vi "Add Hardware.vi"(8 "error in (no error)":errorcluster, 10 "Hardware.lvclass":refnum<class "Hardware.lvclass">, 11 "Controller in":refnum<class "Controller.lvclass">) -> (0 "error out":errorcluster, 3 "Controller out":refnum<class "Controller.lvclass">)   [LabVIEW 2017, in "Controller Actor.lvlib" / "Controller.lvclass"]
uses:
  Controller.lvclass
  C:/Program Files (x86)/National Instruments/LabVIEW 2017/vi.lib/ActorFramework/Actor/Actor.lvclass
  Hardware/Hardware.lvclass
  Controller.lvclass/Controller.ctl
  <userlib>/Configuration Dialog Actor/Configuration.lvclass/Configuration.ctl
  Hardware/Hardware.lvclass/Hardware.ctl
  <vilib>/ActorFramework/Actor/Actor.lvclass/Actor.ctl
  <vilib>/ActorFramework/Message Enqueuer/Message Enqueuer.lvclass/Message Enqueuer.ctl
  <vilib>/ActorFramework/Message Enqueuer/Init from Existing Queue.vi
  Hardware/HW Config/HW Configuration.lvclass
  C:/Program Files (x86)/National Instruments/LabVIEW 2017/user.lib/Configuration Dialog Actor/Configuration.lvclass
  <vilib>/Utility/LVClass/Get LV Class Path.vi
  <userlib>/_OpenG.lib/file/file.llb/Strip Path Extension__ogtk.vi
  <userlib>/_OpenG.lib/file/file.llb/Strip Path Extension - String__ogtk.vi
  <userlib>/Configuration Dialog Actor/Configuration.lvclass
  <vilib>/ActorFramework/Message Enqueuer/Message Enqueuer.lvclass
  Messages/Log Status/Log Status.lvclass
  <vilib>/ActorFramework/Actor/Actor.lvclass
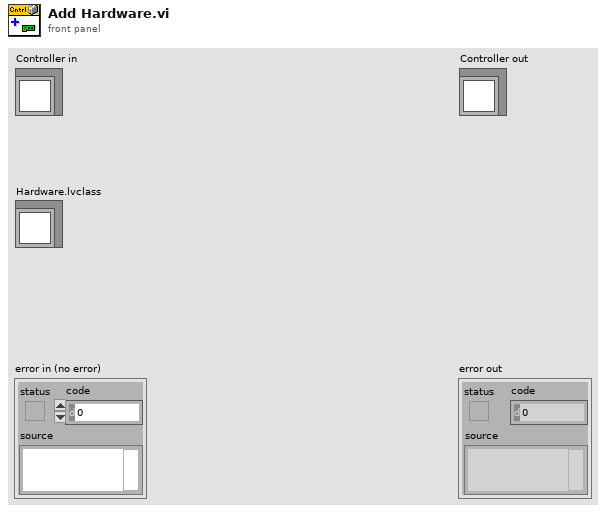
[diagram p1: front panel]
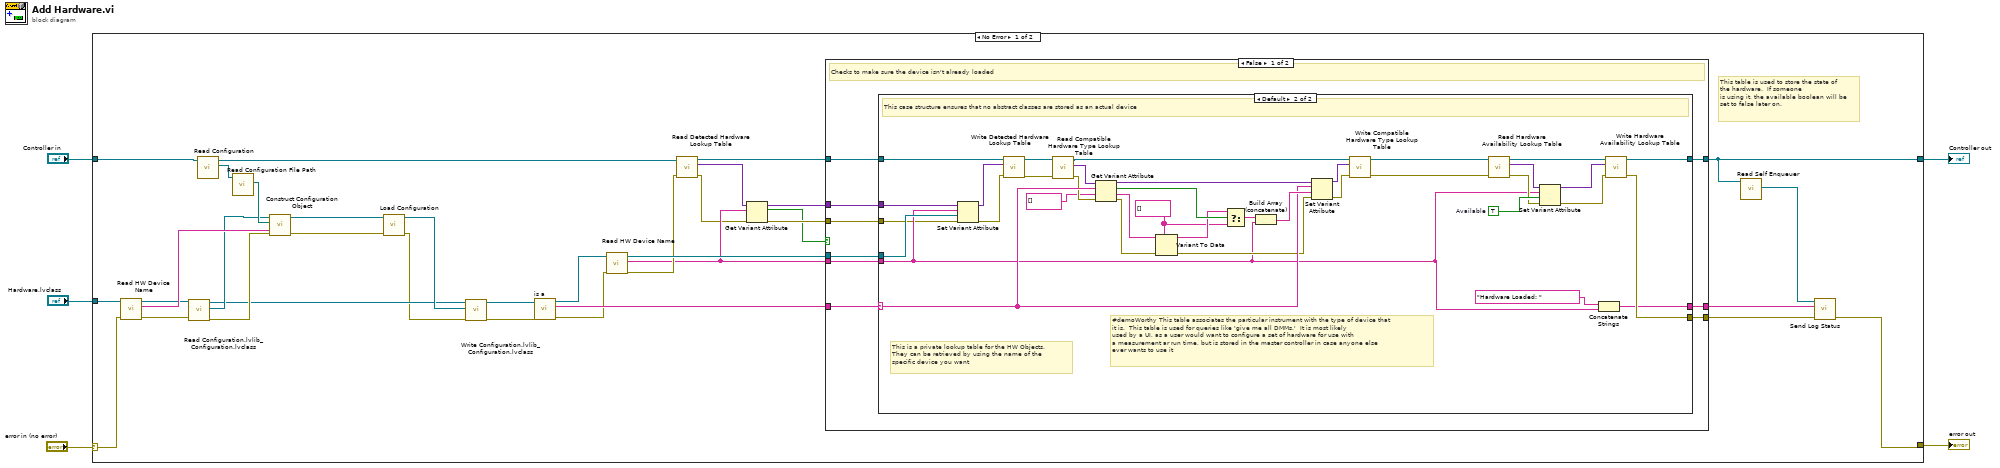
[diagram p0: block diagram]
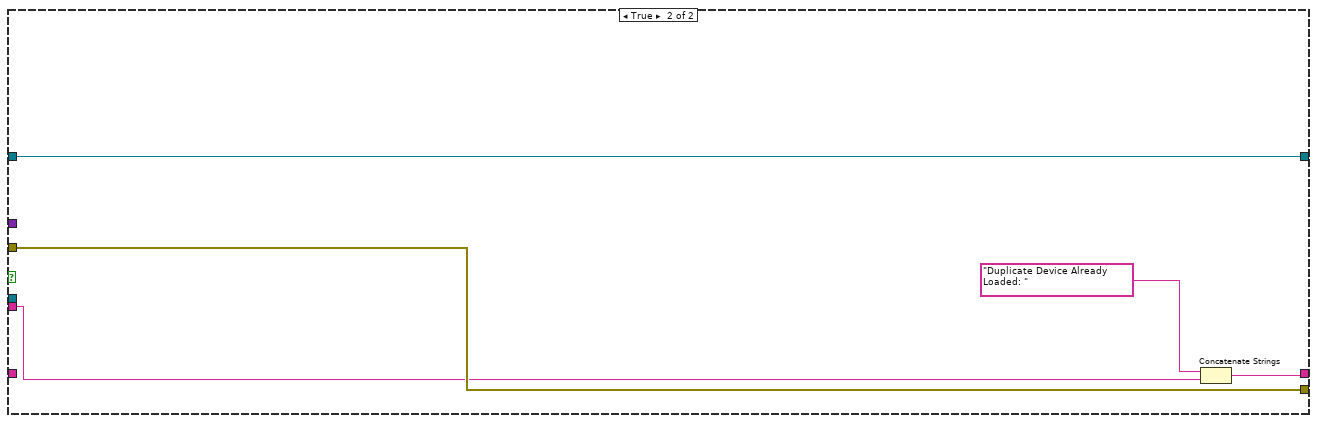
[diagram p3: hidden frame]
diagram:
  n1 = case shown="No Error" "error in (no error)" {
    selector: "error in (no error)" -> [w6 w94]
    tunnel: [w38 w94] -> w4
    tunnel: [w26 w93] -> w2
    tunnel: "Controller in" -> [w19 w93]
    tunnel: "Hardware.lvclass" -> [w17 _]
    frame No Error {
      # "This table is used to store the state of the hardware.  If someone\nis using it, the available boolean will be set to false later on."
      n2 = call "Read HW Device Name.vi"("error in (no error)"=w6, "Analog in"=w17) -> ("error out"=w11:errorcluster, "Device Name"=w16:string, "Analog out"=w13:refnum<class "Hardware.lvclass">)  [unwired: 7 in]
      n3 = call-dynamic "Read Configuration.lvlib_Configuration.lvclass.vi"("error in (no error)"=w11, "Hardware in"=w13) -> ("error out"=w10:errorcluster, "Hardware.lvlib:HW Configuration.lvclass"=w14:refnum<class "HW Configuration.lvclass">, "Hardware out"=w9:refnum<class "Hardware.lvclass">)  [unwired: 7 in]
      n4 = call "Read Configuration.vi"("Controller in"=w19) -> ("Configuration.lvlib:Configuration.lvclass"=w21:refnum<class "Configuration.lvclass">, "Controller out"=w18:refnum<class "Controller.lvclass">)  [unwired: 8 in, 1 out]
      n5 = call <userlib>:"Read Configuration File Path.vi"("Configuration in"=w21) -> ("Configuration File Path"=w20:path)  [unwired: 8 in, 2 out]
      n6 = call <userlib>:"Construct Configuration Object.vi"("Group Name"=w16, "error in (no error)"=w10, "Configuration File Path"=w20, "Configuration in"=w14) -> ("error out"=w22:errorcluster, "Configuration out"=w23:refnum<class "HW Configuration.lvclass">)  [unwired: 4 in, 2 out]
      n7 = call <userlib>:"Load Configuration.vi"("error in (no error)"=w22, "Configuration in"=w23) -> ("error out"=w8:errorcluster, "Configuration out"=w15:refnum<class "HW Configuration.lvclass">)  [unwired: 7 in, 1 out]
      n8 = call-dynamic "Write Configuration.lvlib_Configuration.lvclass.vi"("error in (no error)"=w8, "Hardware.lvlib:HW Configuration.lvclass"=w15, "Hardware in"=w9) -> ("error out"=w7:errorcluster, "Hardware out"=w12:refnum<class "Hardware.lvclass">)  [unwired: 7 in]
      n9 = call-dynamic "is a.vi"("error in (no error)"=w7, "Hardware in"=w12) -> ("error out"=w35:errorcluster, "is a"=w39:string, "Hardware out"=w36:refnum<class "Hardware.lvclass">)  [unwired: 7 in]
      n10 = call "Read HW Device Name.vi"("error in (no error)"=w35, "Analog in"=w36) -> ("error out"=w33:errorcluster, "Device Name"=w30:string, "Analog out"=w37:refnum<class "Hardware.lvclass">)  [unwired: 7 in]
      n11 = call "Read Detected Hardware Lookup Table.vi"("error in (no error)"=w33, "Controller in"=w18) -> ("error out"=w29:errorcluster, "Detected Hardware Lookup Table"=w32:variant, "Controller out"=w34:refnum<class "Controller.lvclass">)  [unwired: 7 in]
      n12 = Get Variant Attribute(Variant=w32, name=w30, error in=w29) -> (duplicate Variant=w31:variant, found=w24:bool, error out=w28:errorcluster)  [unwired: 1 in, 1 out]
      n13 = case shown="False" w24 {
        tunnel: w39 -> [w48 _]
        tunnel: [w47 w91] -> w38
        tunnel: w37 -> [w46 _]
        tunnel: w34 -> [w45 w92]
        tunnel: w31 -> [w44 _]
        tunnel: w30 -> [w43 w88]
        tunnel: w28 -> [w42 w91]
        tunnel: [w41 w92] -> w26
        tunnel: [w40 w89] -> w25
        frame False {
          # "Checks to make sure the device isn't already loaded"
          n14 = case shown="Default" w48 {
            selector: w48 -> [_ w69]
            tunnel: w45 -> [w50 w55]
            tunnel: [w50 w70] -> w41
            tunnel: [w49 w52] -> w47
            tunnel: w46 -> [_ w57]
            tunnel: w43 -> [_ w56]
            tunnel: w44 -> [_ w54]
            tunnel: w42 -> [w49 w53]
            tunnel: [_ w51] -> w40
            frame "Abstract Class" {
            }
            frame Default {
              w75 = TRUE  # Available
              w81 = string[] []
              # "This is a private lookup table for the HW Objects.  \nThey can be retrieved by using the name of the\nspecific device you want"
              # "#demoWorthy This table associates the particular instrument with the type of device that\nit is.  This table is used for queries like 'give me all DMMs.'  It is most likely\nused by a UI, as a user would want to configure a set of hardware for use with\na measurement ar run time, but is stored in the master controller in case anyone else\never wants to use it"
              # "This case structure ensures that no abstract classes are stored as an actual device"
              n15 = Set Variant Attribute(Variant=w54, name=w56, value=w57, error in=w53) -> (Variant out=w87:variant, error out=w66:errorcluster)  [unwired: 1 out]
              n16 = call "Write Detected Hardware Lookup Table.vi"("error in (no error)"=w66, "Detected Hardware Lookup Table"=w87, "Controller in"=w55) -> ("error out"=w67:errorcluster, "Controller out"=w79:refnum<class "Controller.lvclass">)  [unwired: 7 in]
              n17 = call "Read Compatible Hardware Type Lookup Table.vi"("error in (no error)"=w67, "Controller in"=w79) -> ("error out"=w68:errorcluster, "Compatible Hardware Type Lookup Table"=w76:variant, "Controller out"=w78:refnum<class "Controller.lvclass">)  [unwired: 7 in]
              n18 = Get Variant Attribute(Variant=w76, name=w69, default value (empty Variant)=string[] [], error in=w68) -> (duplicate Variant=w80:variant, found=w84:bool, value=w86:string[], error out=w65:errorcluster)
              n19 = Variant To Data(error in=w65, type=w81, Variant=w86) -> (data=w82:string[], error out=w64:errorcluster)
              n20 = Select(t=w82, s=w84, f=w81) -> (s? t:f=w83:string[])
              n21 = Build Array (concatenate)(w83, w56) -> (w85:string[])
              n22 = Set Variant Attribute(Variant=w80, name=w69, value=w85, error in=w64) -> (Variant out=w77:variant, error out=w63:errorcluster)  [unwired: 1 out]
              n23 = call "Write Compatible Hardware Type Lookup Table.vi"("error in (no error)"=w63, "Compatible Hardware Type Lookup Table"=w77, "Controller in"=w78) -> ("error out"=w62:errorcluster, "Controller out"=w74:refnum<class "Controller.lvclass">)  [unwired: 7 in]
              n24 = call "Read Hardware Availability Lookup Table.vi"("error in (no error)"=w62, "Controller in"=w74) -> ("error out"=w61:errorcluster, "Hardware Availability Lookup Table"=w73:variant, "Controller out"=w71:refnum<class "Controller.lvclass">)  [unwired: 7 in]
              n25 = Set Variant Attribute(Variant=w73, name=w56, value=w75, error in=w61) -> (Variant out=w72:variant, error out=w60:errorcluster)  [unwired: 1 out]
              n26 = Concatenate Strings("Hardware Loaded: " ("string"), w56) -> (w51:string)
              n27 = call "Write Hardware Availability Lookup Table.vi"("error in (no error)"=w60, "Hardware Availability Lookup Table"=w72, "Controller in"=w71) -> ("error out"=w52:errorcluster, "Controller out"=w70:refnum<class "Controller.lvclass">)  [unwired: 7 in]
            }
          }
        }
        frame True {
          n28 = Concatenate Strings("Duplicate Device Already Loaded: " ("string"), w88) -> (w89:string)
        }
      }
      n29 = call <vilib>:"Read Self Enqueuer.vi"("Actor"=w26) -> ("Self Enqueuer"=w27:refnum<class "Message Enqueuer.lvclass">)  [unwired: 10 in]
      n30 = call "Send Log Status.vi"("String"=w25, "Message Enqueuer in"=w27) -> ()  [unwired: 8 in, 2 out]
    }
    frame Error {
    }
  }
  "error out" <- w4
  "Controller out" <- w2
